vi "Cronometru cu afisaj 7 segmente.vi"() -> ()   [LabVIEW 2011]
panel:
  out "Boolean 46":bool
  out "Boolean 3":bool
  out "Boolean 2":bool
  out "Boolean":bool
  out "Boolean 45":bool
  out "Boolean 44":bool
  out "Boolean 43":bool
  out "Boolean 42":bool
  out "Boolean 41":bool
  out "Boolean 40":bool
  out "Boolean 39":bool
  out "Boolean 38":bool
  out "Boolean 37":bool
  out "Boolean 36":bool
  out "Boolean 35":bool
  out "Boolean 34":bool
  out "Boolean 33":bool
  out "Boolean 32":bool
  out "Boolean 31":bool
  out "Boolean 30":bool
  out "Boolean 29":bool
  out "Boolean 28":bool
  out "Boolean 27":bool
  out "Boolean 26":bool
  out "Boolean 25":bool
  out "Boolean 24":bool
  out "Boolean 23":bool
  out "Boolean 22":bool
  out "Boolean 21":bool
  out "Boolean 20":bool
  out "Boolean 19":bool
  out "Boolean 18":bool
  out "Boolean 17":bool
  out "Boolean 16":bool
  out "Boolean 15":bool
  out "Boolean 14":bool
  out "Boolean 13":bool
  out "Boolean 12":bool
  out "Boolean 11":bool
  out "Boolean 10":bool
  out "Boolean 9":bool
  out "Boolean 8":bool
  out "Boolean 6":bool
  out "Boolean 7":bool
  out "Boolean 5":bool
  out "Boolean 4":bool
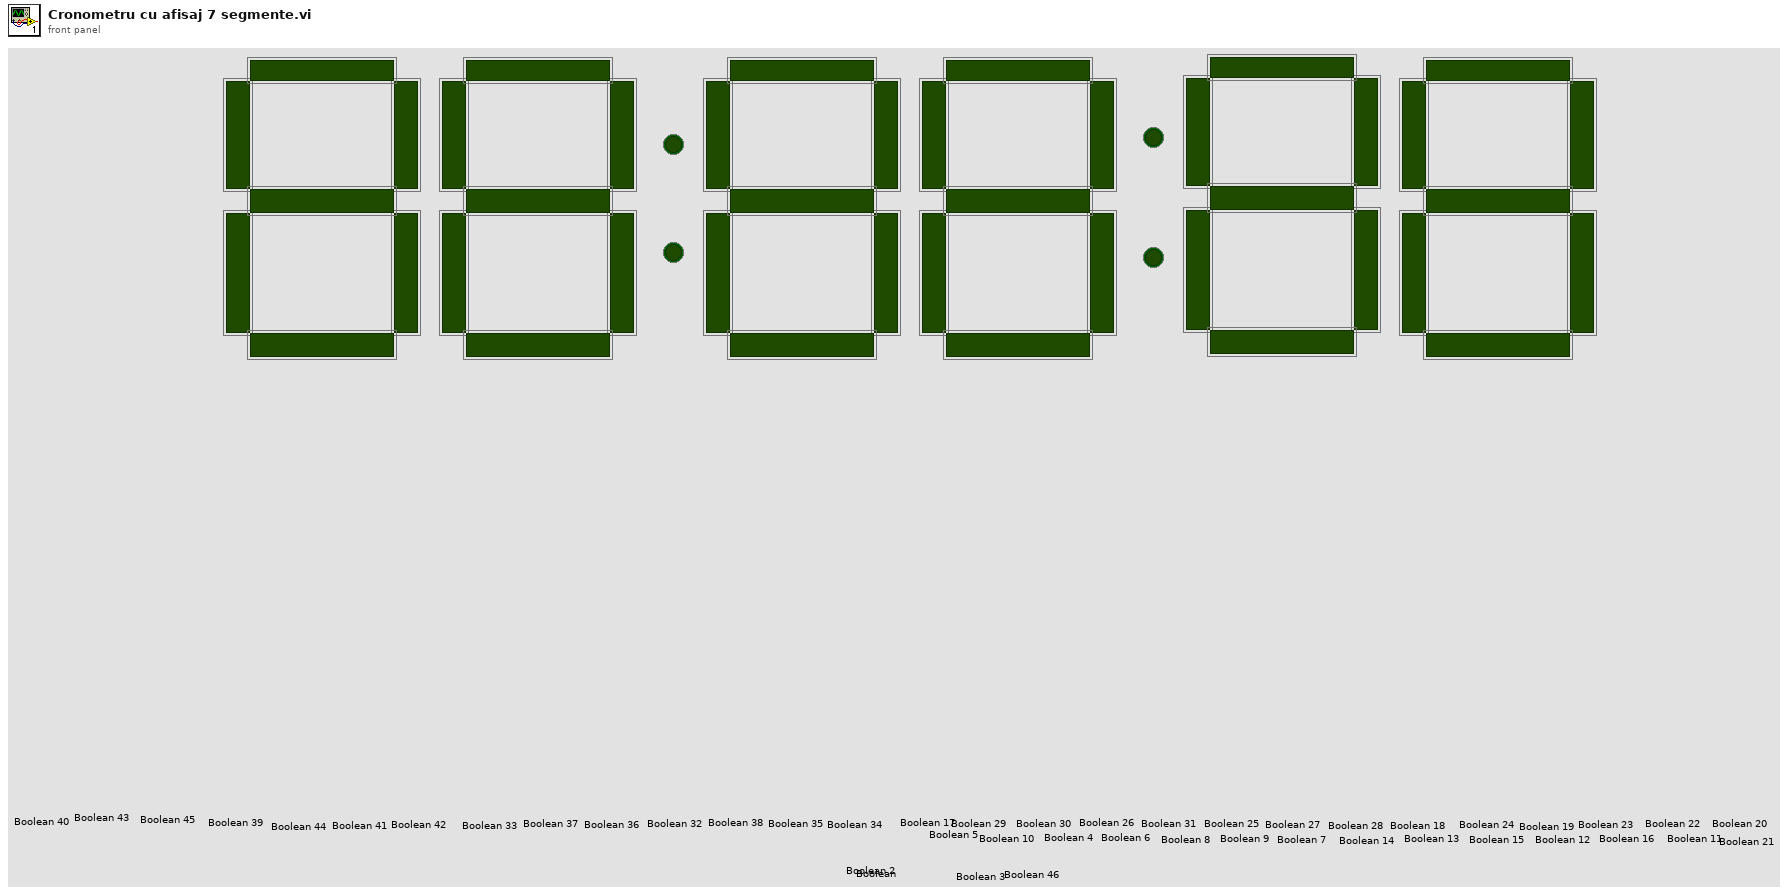
[diagram p1: front panel]
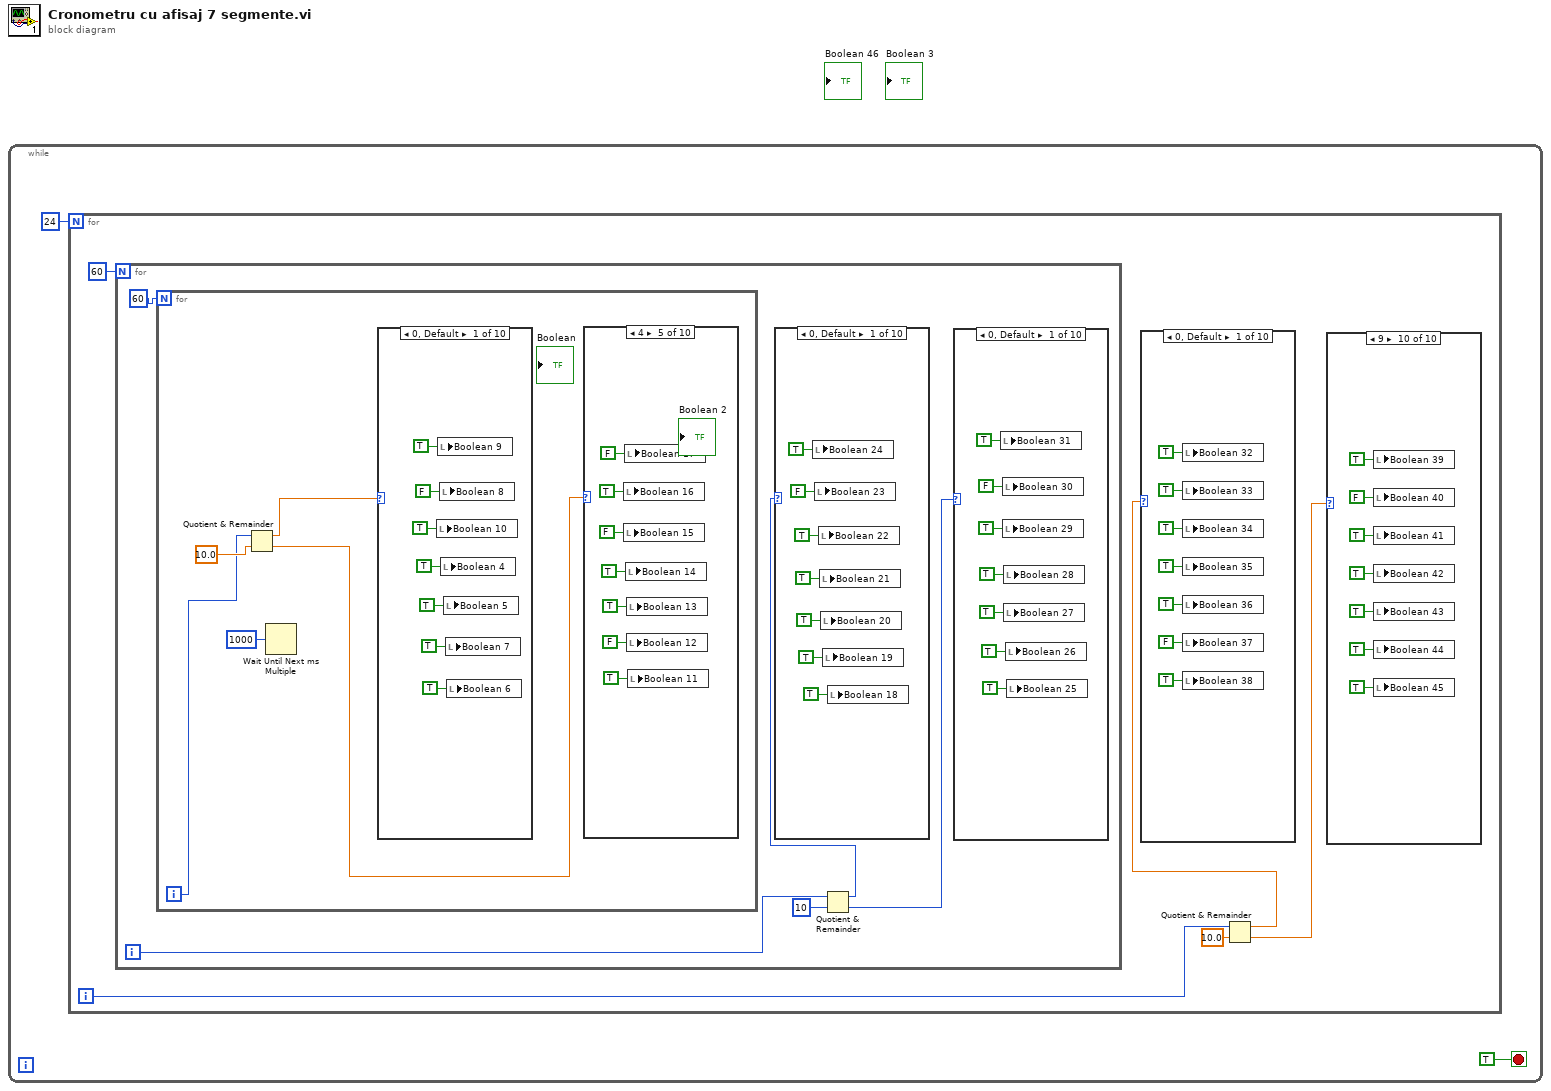
[diagram p0: block diagram]
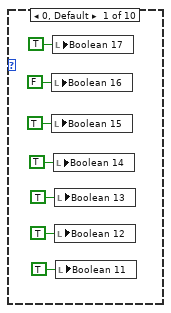
[diagram p2: hidden frame]
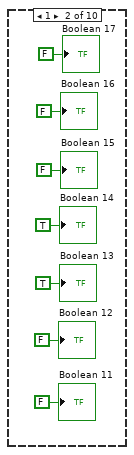
[diagram p3: hidden frame]
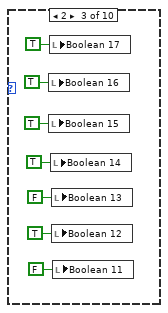
[diagram p4: hidden frame]
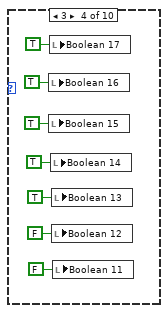
[diagram p5: hidden frame]
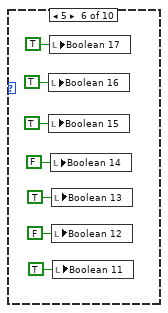
[diagram p6: hidden frame]
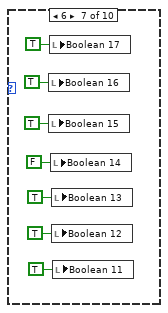
[diagram p7: hidden frame]
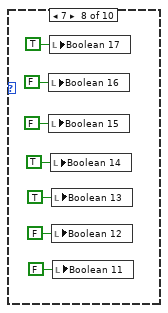
[diagram p8: hidden frame]
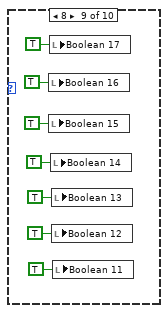
[diagram p9: hidden frame]
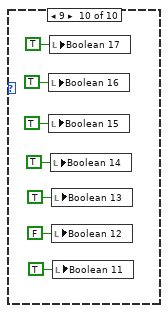
[diagram p10: hidden frame]
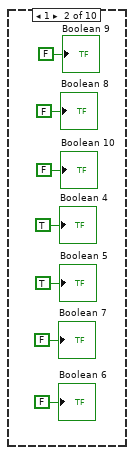
[diagram p11: hidden frame]
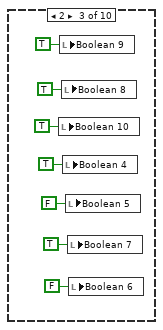
[diagram p12: hidden frame]
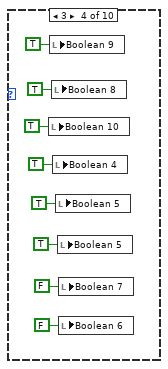
[diagram p13: hidden frame]
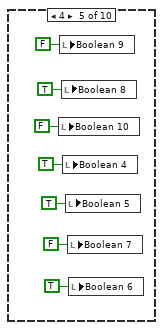
[diagram p14: hidden frame]
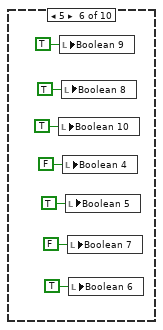
[diagram p15: hidden frame]
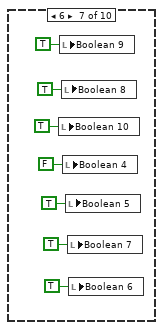
[diagram p16: hidden frame]
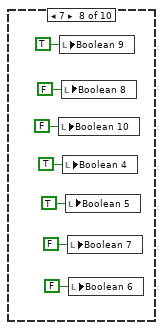
[diagram p17: hidden frame]
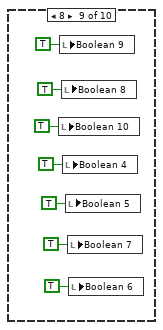
[diagram p18: hidden frame]
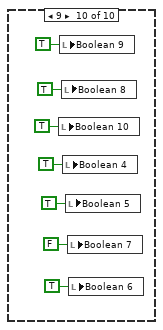
[diagram p19: hidden frame]
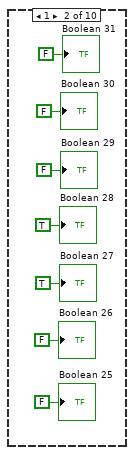
[diagram p20: hidden frame]
diagram:
  n1 = while {
    stop <- TRUE stop-if-true
    n2 = for {
      N: 24 -> [_]
      i -> [w6]
      n3 = for {
        N: 60 -> [_]
        i -> [w11]
        n4 = for {
          N: 60 -> [_]
          i -> [w13]
          n5 = Quotient & Remainder(x=w13, y=10.0 ("x")) -> (x-y*floor(x/y)=w16:dbl, floor(x/y)=w15:dbl)
          n6 = Wait Until Next ms Multiple(millisecond multiple=u32 1000) -> ()  [unwired: 1 out]
          n7 = case shown="0, Default" w16 {
            frame 0, Default {
              n8 = local write "Boolean 10"(TRUE ("Boolean 10")) -> ()
              n9 = local write "Boolean 9"(TRUE ("Boolean 9")) -> ()
              n10 = local write "Boolean 8"(FALSE ("Boolean 8")) -> ()
              n11 = local write "Boolean 4"(TRUE ("Boolean 4")) -> ()
              n12 = local write "Boolean 5"(TRUE ("Boolean 5")) -> ()
              n13 = local write "Boolean 7"(TRUE ("Boolean 5")) -> ()
              n14 = local write "Boolean 6"(TRUE ("Boolean 7")) -> ()
            }
            frame 1 {
              "Boolean 9" <- FALSE ("Boolean 9")
              "Boolean 8" <- FALSE ("Boolean 8")
              "Boolean 10" <- FALSE ("Boolean 10")
              "Boolean 4" <- TRUE ("Boolean 4")
              "Boolean 5" <- TRUE ("Boolean 5")
              "Boolean 7" <- FALSE ("Boolean 7")
              "Boolean 6" <- FALSE ("Boolean 6")
            }
            frame 2 {
              n15 = local write "Boolean 10"(TRUE ("Boolean 10")) -> ()
              n16 = local write "Boolean 9"(TRUE ("Boolean 9")) -> ()
              n17 = local write "Boolean 8"(TRUE ("Boolean 8")) -> ()
              n18 = local write "Boolean 4"(TRUE ("Boolean 4")) -> ()
              n19 = local write "Boolean 5"(FALSE ("Boolean 5")) -> ()
              n20 = local write "Boolean 7"(TRUE ("Boolean 5")) -> ()
              n21 = local write "Boolean 6"(FALSE ("Boolean 7")) -> ()
            }
            frame 3 {
              n22 = local write "Boolean 10"(TRUE ("Boolean 10")) -> ()
              n23 = local write "Boolean 9"(TRUE ("Boolean 9")) -> ()
              n24 = local write "Boolean 8"(TRUE ("Boolean 8")) -> ()
              n25 = local write "Boolean 4"(TRUE ("Boolean 4")) -> ()
              n26 = local write "Boolean 5"(TRUE ("Boolean 5")) -> ()
              n27 = local write "Boolean 5"(TRUE ("Boolean 5")) -> ()
              n28 = local write "Boolean 7"(FALSE ("Boolean 7")) -> ()
              n29 = local write "Boolean 6"(FALSE ("Boolean 6")) -> ()
            }
            frame 4 {
              n30 = local write "Boolean 10"(FALSE ("Boolean 10")) -> ()
              n31 = local write "Boolean 9"(FALSE ("Boolean 9")) -> ()
              n32 = local write "Boolean 8"(TRUE ("Boolean 8")) -> ()
              n33 = local write "Boolean 4"(TRUE ("Boolean 4")) -> ()
              n34 = local write "Boolean 5"(TRUE ("Boolean 5")) -> ()
              n35 = local write "Boolean 7"(FALSE ("Boolean 5")) -> ()
              n36 = local write "Boolean 6"(TRUE ("Boolean 7")) -> ()
            }
            frame 5 {
              n37 = local write "Boolean 10"(TRUE ("Boolean 10")) -> ()
              n38 = local write "Boolean 9"(TRUE ("Boolean 9")) -> ()
              n39 = local write "Boolean 8"(TRUE ("Boolean 8")) -> ()
              n40 = local write "Boolean 4"(FALSE ("Boolean 4")) -> ()
              n41 = local write "Boolean 5"(TRUE ("Boolean 5")) -> ()
              n42 = local write "Boolean 7"(FALSE ("Boolean 5")) -> ()
              n43 = local write "Boolean 6"(TRUE ("Boolean 7")) -> ()
            }
            frame 6 {
              n44 = local write "Boolean 10"(TRUE ("Boolean 10")) -> ()
              n45 = local write "Boolean 9"(TRUE ("Boolean 9")) -> ()
              n46 = local write "Boolean 8"(TRUE ("Boolean 8")) -> ()
              n47 = local write "Boolean 4"(FALSE ("Boolean 4")) -> ()
              n48 = local write "Boolean 5"(TRUE ("Boolean 5")) -> ()
              n49 = local write "Boolean 7"(TRUE ("Boolean 5")) -> ()
              n50 = local write "Boolean 6"(TRUE ("Boolean 7")) -> ()
            }
            frame 7 {
              n51 = local write "Boolean 10"(FALSE ("Boolean 10")) -> ()
              n52 = local write "Boolean 9"(TRUE ("Boolean 9")) -> ()
              n53 = local write "Boolean 8"(FALSE ("Boolean 8")) -> ()
              n54 = local write "Boolean 4"(TRUE ("Boolean 4")) -> ()
              n55 = local write "Boolean 5"(TRUE ("Boolean 5")) -> ()
              n56 = local write "Boolean 7"(FALSE ("Boolean 5")) -> ()
              n57 = local write "Boolean 6"(FALSE ("Boolean 7")) -> ()
            }
            frame 8 {
              n58 = local write "Boolean 10"(TRUE ("Boolean 10")) -> ()
              n59 = local write "Boolean 9"(TRUE ("Boolean 9")) -> ()
              n60 = local write "Boolean 8"(TRUE ("Boolean 8")) -> ()
              n61 = local write "Boolean 4"(TRUE ("Boolean 4")) -> ()
              n62 = local write "Boolean 5"(TRUE ("Boolean 5")) -> ()
              n63 = local write "Boolean 7"(TRUE ("Boolean 5")) -> ()
              n64 = local write "Boolean 6"(TRUE ("Boolean 7")) -> ()
            }
            frame 9 {
              n65 = local write "Boolean 10"(TRUE ("Boolean 10")) -> ()
              n66 = local write "Boolean 9"(TRUE ("Boolean 9")) -> ()
              n67 = local write "Boolean 8"(TRUE ("Boolean 8")) -> ()
              n68 = local write "Boolean 4"(TRUE ("Boolean 4")) -> ()
              n69 = local write "Boolean 5"(TRUE ("Boolean 5")) -> ()
              n70 = local write "Boolean 7"(FALSE ("Boolean 5")) -> ()
              n71 = local write "Boolean 6"(TRUE ("Boolean 7")) -> ()
            }
          }
          n72 = case shown="4" w15 {
            frame 0, Default {
              n73 = local write "Boolean 16"(FALSE ("Boolean 16")) -> ()
              n74 = local write "Boolean 15"(TRUE ("Boolean 15")) -> ()
              n75 = local write "Boolean 17"(TRUE ("Boolean 17")) -> ()
              n76 = local write "Boolean 14"(TRUE ("Boolean 14")) -> ()
              n77 = local write "Boolean 13"(TRUE ("Boolean 13")) -> ()
              n78 = local write "Boolean 12"(TRUE ("Boolean 12")) -> ()
              n79 = local write "Boolean 11"(TRUE ("Boolean 11")) -> ()
            }
            frame 1 {
              "Boolean 17" <- FALSE ("Boolean 9")
              "Boolean 16" <- FALSE ("Boolean 8")
              "Boolean 15" <- FALSE ("Boolean 10")
              "Boolean 14" <- TRUE ("Boolean 4")
              "Boolean 13" <- TRUE ("Boolean 5")
              "Boolean 12" <- FALSE ("Boolean 7")
              "Boolean 11" <- FALSE ("Boolean 6")
            }
            frame 2 {
              n80 = local write "Boolean 16"(TRUE ("Boolean 16")) -> ()
              n81 = local write "Boolean 15"(TRUE ("Boolean 15")) -> ()
              n82 = local write "Boolean 17"(TRUE ("Boolean 17")) -> ()
              n83 = local write "Boolean 14"(TRUE ("Boolean 14")) -> ()
              n84 = local write "Boolean 13"(FALSE ("Boolean 13")) -> ()
              n85 = local write "Boolean 12"(TRUE ("Boolean 12")) -> ()
              n86 = local write "Boolean 11"(FALSE ("Boolean 11")) -> ()
            }
            frame 3 {
              n87 = local write "Boolean 16"(TRUE ("Boolean 16")) -> ()
              n88 = local write "Boolean 15"(TRUE ("Boolean 15")) -> ()
              n89 = local write "Boolean 17"(TRUE ("Boolean 17")) -> ()
              n90 = local write "Boolean 14"(TRUE ("Boolean 14")) -> ()
              n91 = local write "Boolean 13"(TRUE ("Boolean 13")) -> ()
              n92 = local write "Boolean 12"(FALSE ("Boolean 12")) -> ()
              n93 = local write "Boolean 11"(FALSE ("Boolean 11")) -> ()
            }
            frame 4 {
              n94 = local write "Boolean 16"(TRUE ("Boolean 16")) -> ()
              n95 = local write "Boolean 15"(FALSE ("Boolean 15")) -> ()
              n96 = local write "Boolean 17"(FALSE ("Boolean 17")) -> ()
              n97 = local write "Boolean 14"(TRUE ("Boolean 14")) -> ()
              n98 = local write "Boolean 13"(TRUE ("Boolean 13")) -> ()
              n99 = local write "Boolean 12"(FALSE ("Boolean 12")) -> ()
              n100 = local write "Boolean 11"(TRUE ("Boolean 11")) -> ()
            }
            frame 5 {
              n101 = local write "Boolean 16"(TRUE ("Boolean 16")) -> ()
              n102 = local write "Boolean 15"(TRUE ("Boolean 15")) -> ()
              n103 = local write "Boolean 17"(TRUE ("Boolean 17")) -> ()
              n104 = local write "Boolean 14"(FALSE ("Boolean 14")) -> ()
              n105 = local write "Boolean 13"(TRUE ("Boolean 13")) -> ()
              n106 = local write "Boolean 12"(FALSE ("Boolean 12")) -> ()
              n107 = local write "Boolean 11"(TRUE ("Boolean 11")) -> ()
            }
            frame 6 {
              n108 = local write "Boolean 16"(TRUE ("Boolean 16")) -> ()
              n109 = local write "Boolean 15"(TRUE ("Boolean 15")) -> ()
              n110 = local write "Boolean 17"(TRUE ("Boolean 17")) -> ()
              n111 = local write "Boolean 14"(FALSE ("Boolean 14")) -> ()
              n112 = local write "Boolean 13"(TRUE ("Boolean 13")) -> ()
              n113 = local write "Boolean 12"(TRUE ("Boolean 12")) -> ()
              n114 = local write "Boolean 11"(TRUE ("Boolean 11")) -> ()
            }
            frame 7 {
              n115 = local write "Boolean 16"(FALSE ("Boolean 16")) -> ()
              n116 = local write "Boolean 15"(FALSE ("Boolean 15")) -> ()
              n117 = local write "Boolean 17"(TRUE ("Boolean 17")) -> ()
              n118 = local write "Boolean 14"(TRUE ("Boolean 14")) -> ()
              n119 = local write "Boolean 13"(TRUE ("Boolean 13")) -> ()
              n120 = local write "Boolean 12"(FALSE ("Boolean 12")) -> ()
              n121 = local write "Boolean 11"(FALSE ("Boolean 11")) -> ()
            }
            frame 8 {
              n122 = local write "Boolean 16"(TRUE ("Boolean 16")) -> ()
              n123 = local write "Boolean 15"(TRUE ("Boolean 15")) -> ()
              n124 = local write "Boolean 17"(TRUE ("Boolean 17")) -> ()
              n125 = local write "Boolean 14"(TRUE ("Boolean 14")) -> ()
              n126 = local write "Boolean 13"(TRUE ("Boolean 13")) -> ()
              n127 = local write "Boolean 12"(TRUE ("Boolean 12")) -> ()
              n128 = local write "Boolean 11"(TRUE ("Boolean 11")) -> ()
            }
            frame 9 {
              n129 = local write "Boolean 16"(TRUE ("Boolean 16")) -> ()
              n130 = local write "Boolean 15"(TRUE ("Boolean 15")) -> ()
              n131 = local write "Boolean 17"(TRUE ("Boolean 17")) -> ()
              n132 = local write "Boolean 14"(TRUE ("Boolean 14")) -> ()
              n133 = local write "Boolean 13"(TRUE ("Boolean 13")) -> ()
              n134 = local write "Boolean 12"(FALSE ("Boolean 12")) -> ()
              n135 = local write "Boolean 11"(TRUE ("Boolean 11")) -> ()
            }
          }
        }
        n136 = Quotient & Remainder(x=w11, y=10) -> (x-y*floor(x/y)=w9:i32, floor(x/y)=w8:i32)
        n137 = case shown="0, Default" w9 {
          frame 0, Default {
            n138 = local write "Boolean 24"(TRUE ("Boolean 24")) -> ()
            n139 = local write "Boolean 23"(FALSE ("Boolean 23")) -> ()
            n140 = local write "Boolean 22"(TRUE ("Boolean 22")) -> ()
            n141 = local write "Boolean 21"(TRUE ("Boolean 21")) -> ()
            n142 = local write "Boolean 20"(TRUE ("Boolean 20")) -> ()
            n143 = local write "Boolean 19"(TRUE ("Boolean 19")) -> ()
            n144 = local write "Boolean 18"(TRUE ("Boolean 18")) -> ()
          }
          frame 1 {
            "Boolean 24" <- FALSE ("Boolean 9")
            "Boolean 23" <- FALSE ("Boolean 8")
            "Boolean 22" <- FALSE ("Boolean 10")
            "Boolean 21" <- TRUE ("Boolean 4")
            "Boolean 20" <- TRUE ("Boolean 5")
            "Boolean 19" <- FALSE ("Boolean 7")
            "Boolean 18" <- FALSE ("Boolean 6")
          }
          frame 2 {
            n145 = local write "Boolean 24"(TRUE ("Boolean 24")) -> ()
            n146 = local write "Boolean 23"(TRUE ("Boolean 23")) -> ()
            n147 = local write "Boolean 22"(TRUE ("Boolean 22")) -> ()
            n148 = local write "Boolean 21"(TRUE ("Boolean 21")) -> ()
            n149 = local write "Boolean 20"(FALSE ("Boolean 20")) -> ()
            n150 = local write "Boolean 19"(TRUE ("Boolean 19")) -> ()
            n151 = local write "Boolean 18"(FALSE ("Boolean 18")) -> ()
          }
          frame 3 {
            n152 = local write "Boolean 24"(TRUE ("Boolean 24")) -> ()
            n153 = local write "Boolean 23"(TRUE ("Boolean 23")) -> ()
            n154 = local write "Boolean 22"(TRUE ("Boolean 22")) -> ()
            n155 = local write "Boolean 21"(TRUE ("Boolean 21")) -> ()
            n156 = local write "Boolean 20"(TRUE ("Boolean 20")) -> ()
            n157 = local write "Boolean 19"(FALSE ("Boolean 19")) -> ()
            n158 = local write "Boolean 18"(FALSE ("Boolean 18")) -> ()
          }
          frame 4 {
            n159 = local write "Boolean 24"(FALSE ("Boolean 24")) -> ()
            n160 = local write "Boolean 23"(TRUE ("Boolean 23")) -> ()
            n161 = local write "Boolean 22"(FALSE ("Boolean 22")) -> ()
            n162 = local write "Boolean 21"(TRUE ("Boolean 21")) -> ()
            n163 = local write "Boolean 20"(TRUE ("Boolean 20")) -> ()
            n164 = local write "Boolean 19"(FALSE ("Boolean 19")) -> ()
            n165 = local write "Boolean 18"(TRUE ("Boolean 18")) -> ()
          }
          frame 5 {
            n166 = local write "Boolean 24"(TRUE ("Boolean 24")) -> ()
            n167 = local write "Boolean 23"(TRUE ("Boolean 23")) -> ()
            n168 = local write "Boolean 22"(TRUE ("Boolean 22")) -> ()
            n169 = local write "Boolean 21"(FALSE ("Boolean 21")) -> ()
            n170 = local write "Boolean 20"(TRUE ("Boolean 20")) -> ()
            n171 = local write "Boolean 19"(FALSE ("Boolean 19")) -> ()
            n172 = local write "Boolean 18"(TRUE ("Boolean 18")) -> ()
          }
          frame 6 {
            n173 = local write "Boolean 24"(TRUE ("Boolean 24")) -> ()
            n174 = local write "Boolean 23"(TRUE ("Boolean 23")) -> ()
            n175 = local write "Boolean 22"(TRUE ("Boolean 22")) -> ()
            n176 = local write "Boolean 21"(FALSE ("Boolean 21")) -> ()
            n177 = local write "Boolean 20"(TRUE ("Boolean 20")) -> ()
            n178 = local write "Boolean 19"(TRUE ("Boolean 19")) -> ()
            n179 = local write "Boolean 18"(TRUE ("Boolean 18")) -> ()
          }
          frame 7 {
            n180 = local write "Boolean 24"(TRUE ("Boolean 24")) -> ()
            n181 = local write "Boolean 23"(FALSE ("Boolean 23")) -> ()
            n182 = local write "Boolean 22"(FALSE ("Boolean 22")) -> ()
            n183 = local write "Boolean 21"(TRUE ("Boolean 21")) -> ()
            n184 = local write "Boolean 20"(TRUE ("Boolean 20")) -> ()
            n185 = local write "Boolean 19"(FALSE ("Boolean 19")) -> ()
            n186 = local write "Boolean 18"(FALSE ("Boolean 18")) -> ()
          }
          frame 8 {
            n187 = local write "Boolean 24"(TRUE ("Boolean 24")) -> ()
            n188 = local write "Boolean 23"(TRUE ("Boolean 23")) -> ()
            n189 = local write "Boolean 22"(TRUE ("Boolean 22")) -> ()
            n190 = local write "Boolean 21"(TRUE ("Boolean 21")) -> ()
            n191 = local write "Boolean 20"(TRUE ("Boolean 20")) -> ()
            n192 = local write "Boolean 19"(TRUE ("Boolean 19")) -> ()
            n193 = local write "Boolean 18"(TRUE ("Boolean 18")) -> ()
          }
          frame 9 {
            n194 = local write "Boolean 24"(TRUE ("Boolean 24")) -> ()
            n195 = local write "Boolean 23"(TRUE ("Boolean 23")) -> ()
            n196 = local write "Boolean 22"(TRUE ("Boolean 22")) -> ()
            n197 = local write "Boolean 21"(TRUE ("Boolean 21")) -> ()
            n198 = local write "Boolean 20"(TRUE ("Boolean 20")) -> ()
            n199 = local write "Boolean 19"(FALSE ("Boolean 19")) -> ()
            n200 = local write "Boolean 18"(TRUE ("Boolean 18")) -> ()
          }
        }
        n201 = case shown="0, Default" w8 {
          frame 0, Default {
            n202 = local write "Boolean 31"(TRUE ("Boolean 31")) -> ()
            n203 = local write "Boolean 30"(FALSE ("Boolean 30")) -> ()
            n204 = local write "Boolean 29"(TRUE ("Boolean 29")) -> ()
            n205 = local write "Boolean 28"(TRUE ("Boolean 28")) -> ()
            n206 = local write "Boolean 27"(TRUE ("Boolean 27")) -> ()
            n207 = local write "Boolean 26"(TRUE ("Boolean 26")) -> ()
            n208 = local write "Boolean 25"(TRUE ("Boolean 25")) -> ()
          }
          frame 1 {
            "Boolean 31" <- FALSE ("Boolean 9")
            "Boolean 30" <- FALSE ("Boolean 8")
            "Boolean 29" <- FALSE ("Boolean 10")
            "Boolean 28" <- TRUE ("Boolean 4")
            "Boolean 27" <- TRUE ("Boolean 5")
            "Boolean 26" <- FALSE ("Boolean 7")
            "Boolean 25" <- FALSE ("Boolean 6")
          }
          frame 2 {
            n209 = local write "Boolean 31"(TRUE ("Boolean 31")) -> ()
            n210 = local write "Boolean 30"(TRUE ("Boolean 30")) -> ()
            n211 = local write "Boolean 29"(TRUE ("Boolean 29")) -> ()
            n212 = local write "Boolean 28"(TRUE ("Boolean 28")) -> ()
            n213 = local write "Boolean 27"(FALSE ("Boolean 27")) -> ()
            n214 = local write "Boolean 26"(TRUE ("Boolean 26")) -> ()
            n215 = local write "Boolean 25"(FALSE ("Boolean 25")) -> ()
          }
          frame 3 {
            n216 = local write "Boolean 31"(TRUE ("Boolean 31")) -> ()
            n217 = local write "Boolean 30"(TRUE ("Boolean 30")) -> ()
            n218 = local write "Boolean 29"(TRUE ("Boolean 29")) -> ()
            n219 = local write "Boolean 28"(TRUE ("Boolean 28")) -> ()
            n220 = local write "Boolean 27"(TRUE ("Boolean 27")) -> ()
            n221 = local write "Boolean 26"(FALSE ("Boolean 26")) -> ()
            n222 = local write "Boolean 25"(FALSE ("Boolean 25")) -> ()
          }
          frame 4 {
            n223 = local write "Boolean 31"(FALSE ("Boolean 31")) -> ()
            n224 = local write "Boolean 30"(TRUE ("Boolean 30")) -> ()
            n225 = local write "Boolean 29"(FALSE ("Boolean 29")) -> ()
            n226 = local write "Boolean 28"(TRUE ("Boolean 28")) -> ()
            n227 = local write "Boolean 27"(TRUE ("Boolean 27")) -> ()
            n228 = local write "Boolean 26"(FALSE ("Boolean 26")) -> ()
            n229 = local write "Boolean 25"(TRUE ("Boolean 25")) -> ()
          }
          frame 5 {
            n230 = local write "Boolean 31"(TRUE ("Boolean 31")) -> ()
            n231 = local write "Boolean 30"(TRUE ("Boolean 30")) -> ()
            n232 = local write "Boolean 29"(TRUE ("Boolean 29")) -> ()
            n233 = local write "Boolean 28"(FALSE ("Boolean 28")) -> ()
            n234 = local write "Boolean 27"(TRUE ("Boolean 27")) -> ()
            n235 = local write "Boolean 26"(FALSE ("Boolean 26")) -> ()
            n236 = local write "Boolean 25"(TRUE ("Boolean 25")) -> ()
          }
          frame 6 {
            n237 = local write "Boolean 31"(TRUE ("Boolean 31")) -> ()
            n238 = local write "Boolean 30"(TRUE ("Boolean 30")) -> ()
            n239 = local write "Boolean 29"(TRUE ("Boolean 29")) -> ()
            n240 = local write "Boolean 28"(FALSE ("Boolean 28")) -> ()
            n241 = local write "Boolean 27"(TRUE ("Boolean 27")) -> ()
            n242 = local write "Boolean 26"(TRUE ("Boolean 26")) -> ()
            n243 = local write "Boolean 25"(TRUE ("Boolean 25")) -> ()
          }
          frame 7 {
            n244 = local write "Boolean 31"(TRUE ("Boolean 31")) -> ()
            n245 = local write "Boolean 30"(FALSE ("Boolean 30")) -> ()
            n246 = local write "Boolean 29"(FALSE ("Boolean 29")) -> ()
            n247 = local write "Boolean 28"(TRUE ("Boolean 28")) -> ()
            n248 = local write "Boolean 27"(TRUE ("Boolean 27")) -> ()
            n249 = local write "Boolean 26"(FALSE ("Boolean 26")) -> ()
            n250 = local write "Boolean 25"(FALSE ("Boolean 25")) -> ()
          }
          frame 8 {
            n251 = local write "Boolean 31"(TRUE ("Boolean 31")) -> ()
            n252 = local write "Boolean 30"(TRUE ("Boolean 30")) -> ()
            n253 = local write "Boolean 29"(TRUE ("Boolean 29")) -> ()
            n254 = local write "Boolean 28"(TRUE ("Boolean 28")) -> ()
            n255 = local write "Boolean 27"(TRUE ("Boolean 27")) -> ()
            n256 = local write "Boolean 26"(TRUE ("Boolean 26")) -> ()
            n257 = local write "Boolean 25"(TRUE ("Boolean 25")) -> ()
          }
          frame 9 {
            n258 = local write "Boolean 31"(TRUE ("Boolean 31")) -> ()
            n259 = local write "Boolean 30"(TRUE ("Boolean 30")) -> ()
            n260 = local write "Boolean 29"(TRUE ("Boolean 29")) -> ()
            n261 = local write "Boolean 28"(TRUE ("Boolean 28")) -> ()
            n262 = local write "Boolean 27"(TRUE ("Boolean 27")) -> ()
            n263 = local write "Boolean 26"(FALSE ("Boolean 26")) -> ()
            n264 = local write "Boolean 25"(TRUE ("Boolean 25")) -> ()
          }
        }
      }
      n265 = Quotient & Remainder(x=w6, y=10.0 ("floor(x/y)")) -> (x-y*floor(x/y)=w5:dbl, floor(x/y)=w4:dbl)
      n266 = case shown="0, Default" w5 {
        frame 0, Default {
          n267 = local write "Boolean 32"(TRUE ("Boolean 32")) -> ()
          n268 = local write "Boolean 33"(TRUE ("Boolean 33")) -> ()
          n269 = local write "Boolean 34"(TRUE ("Boolean 34")) -> ()
          n270 = local write "Boolean 35"(TRUE ("Boolean 35")) -> ()
          n271 = local write "Boolean 36"(TRUE ("Boolean 36")) -> ()
          n272 = local write "Boolean 37"(FALSE ("Boolean 37")) -> ()
          n273 = local write "Boolean 38"(TRUE ("Boolean 38")) -> ()
        }
        frame 1 {
          "Boolean 38" <- FALSE ("Boolean 9")
          "Boolean 37" <- FALSE ("Boolean 8")
          "Boolean 36" <- FALSE ("Boolean 10")
          "Boolean 35" <- TRUE ("Boolean 4")
          "Boolean 34" <- TRUE ("Boolean 5")
          "Boolean 33" <- FALSE ("Boolean 7")
          "Boolean 32" <- FALSE ("Boolean 6")
        }
        frame 2 {
          n274 = local write "Boolean 32"(FALSE ("Boolean 32")) -> ()
          n275 = local write "Boolean 33"(TRUE ("Boolean 33")) -> ()
          n276 = local write "Boolean 34"(FALSE ("Boolean 34")) -> ()
          n277 = local write "Boolean 35"(TRUE ("Boolean 35")) -> ()
          n278 = local write "Boolean 36"(TRUE ("Boolean 36")) -> ()
          n279 = local write "Boolean 37"(TRUE ("Boolean 37")) -> ()
          n280 = local write "Boolean 38"(TRUE ("Boolean 38")) -> ()
        }
        frame 3 {
          n281 = local write "Boolean 32"(FALSE ("Boolean 32")) -> ()
          n282 = local write "Boolean 33"(FALSE ("Boolean 33")) -> ()
          n283 = local write "Boolean 34"(TRUE ("Boolean 34")) -> ()
          n284 = local write "Boolean 35"(TRUE ("Boolean 35")) -> ()
          n285 = local write "Boolean 36"(TRUE ("Boolean 36")) -> ()
          n286 = local write "Boolean 37"(TRUE ("Boolean 37")) -> ()
          n287 = local write "Boolean 38"(TRUE ("Boolean 38")) -> ()
        }
        frame 4 {
          n288 = local write "Boolean 32"(TRUE ("Boolean 32")) -> ()
          n289 = local write "Boolean 33"(FALSE ("Boolean 33")) -> ()
          n290 = local write "Boolean 34"(TRUE ("Boolean 34")) -> ()
          n291 = local write "Boolean 35"(TRUE ("Boolean 35")) -> ()
          n292 = local write "Boolean 36"(FALSE ("Boolean 36")) -> ()
          n293 = local write "Boolean 37"(TRUE ("Boolean 37")) -> ()
          n294 = local write "Boolean 38"(FALSE ("Boolean 38")) -> ()
        }
        frame 5 {
          n295 = local write "Boolean 32"(TRUE ("Boolean 32")) -> ()
          n296 = local write "Boolean 33"(FALSE ("Boolean 33")) -> ()
          n297 = local write "Boolean 34"(TRUE ("Boolean 34")) -> ()
          n298 = local write "Boolean 35"(FALSE ("Boolean 35")) -> ()
          n299 = local write "Boolean 36"(TRUE ("Boolean 36")) -> ()
          n300 = local write "Boolean 37"(TRUE ("Boolean 37")) -> ()
          n301 = local write "Boolean 38"(TRUE ("Boolean 38")) -> ()
        }
        frame 6 {
          n302 = local write "Boolean 32"(TRUE ("Boolean 32")) -> ()
          n303 = local write "Boolean 33"(TRUE ("Boolean 33")) -> ()
          n304 = local write "Boolean 34"(TRUE ("Boolean 34")) -> ()
          n305 = local write "Boolean 35"(FALSE ("Boolean 35")) -> ()
          n306 = local write "Boolean 36"(TRUE ("Boolean 36")) -> ()
          n307 = local write "Boolean 37"(TRUE ("Boolean 37")) -> ()
          n308 = local write "Boolean 38"(TRUE ("Boolean 38")) -> ()
        }
        frame 7 {
          n309 = local write "Boolean 32"(FALSE ("Boolean 32")) -> ()
          n310 = local write "Boolean 33"(FALSE ("Boolean 33")) -> ()
          n311 = local write "Boolean 34"(TRUE ("Boolean 34")) -> ()
          n312 = local write "Boolean 35"(TRUE ("Boolean 35")) -> ()
          n313 = local write "Boolean 36"(FALSE ("Boolean 36")) -> ()
          n314 = local write "Boolean 37"(FALSE ("Boolean 37")) -> ()
          n315 = local write "Boolean 38"(TRUE ("Boolean 38")) -> ()
        }
        frame 8 {
          n316 = local write "Boolean 32"(TRUE ("Boolean 32")) -> ()
          n317 = local write "Boolean 33"(TRUE ("Boolean 33")) -> ()
          n318 = local write "Boolean 34"(TRUE ("Boolean 34")) -> ()
          n319 = local write "Boolean 35"(TRUE ("Boolean 35")) -> ()
          n320 = local write "Boolean 36"(TRUE ("Boolean 36")) -> ()
          n321 = local write "Boolean 37"(TRUE ("Boolean 37")) -> ()
          n322 = local write "Boolean 38"(TRUE ("Boolean 38")) -> ()
        }
        frame 9 {
          n323 = local write "Boolean 32"(TRUE ("Boolean 32")) -> ()
          n324 = local write "Boolean 33"(FALSE ("Boolean 33")) -> ()
          n325 = local write "Boolean 34"(TRUE ("Boolean 34")) -> ()
          n326 = local write "Boolean 35"(TRUE ("Boolean 35")) -> ()
          n327 = local write "Boolean 36"(TRUE ("Boolean 36")) -> ()
          n328 = local write "Boolean 37"(TRUE ("Boolean 37")) -> ()
          n329 = local write "Boolean 38"(TRUE ("Boolean 38")) -> ()
        }
      }
      n330 = case shown="9" w4 {
        frame 0, Default {
          n331 = local write "Boolean 39"(TRUE ("Boolean 39")) -> ()
          n332 = local write "Boolean 40"(TRUE ("Boolean 40")) -> ()
          n333 = local write "Boolean 41"(TRUE ("Boolean 41")) -> ()
          n334 = local write "Boolean 42"(TRUE ("Boolean 42")) -> ()
          n335 = local write "Boolean 43"(TRUE ("Boolean 43")) -> ()
          n336 = local write "Boolean 44"(FALSE ("Boolean 44")) -> ()
          n337 = local write "Boolean 45"(TRUE ("Boolean 45")) -> ()
        }
        frame 1 {
          "Boolean 45" <- FALSE ("Boolean 9")
          "Boolean 44" <- FALSE ("Boolean 8")
          "Boolean 43" <- FALSE ("Boolean 10")
          "Boolean 42" <- TRUE ("Boolean 4")
          "Boolean 41" <- TRUE ("Boolean 5")
          "Boolean 40" <- FALSE ("Boolean 7")
          "Boolean 39" <- FALSE ("Boolean 6")
        }
        frame 2 {
          n338 = local write "Boolean 39"(FALSE ("Boolean 39")) -> ()
          n339 = local write "Boolean 40"(TRUE ("Boolean 40")) -> ()
          n340 = local write "Boolean 41"(FALSE ("Boolean 41")) -> ()
          n341 = local write "Boolean 42"(TRUE ("Boolean 42")) -> ()
          n342 = local write "Boolean 43"(TRUE ("Boolean 43")) -> ()
          n343 = local write "Boolean 44"(TRUE ("Boolean 44")) -> ()
          n344 = local write "Boolean 45"(TRUE ("Boolean 45")) -> ()
        }
        frame 3 {
          n345 = local write "Boolean 39"(FALSE ("Boolean 39")) -> ()
          n346 = local write "Boolean 40"(FALSE ("Boolean 40")) -> ()
          n347 = local write "Boolean 41"(TRUE ("Boolean 41")) -> ()
          n348 = local write "Boolean 42"(TRUE ("Boolean 42")) -> ()
          n349 = local write "Boolean 43"(TRUE ("Boolean 43")) -> ()
          n350 = local write "Boolean 44"(TRUE ("Boolean 44")) -> ()
          n351 = local write "Boolean 45"(TRUE ("Boolean 45")) -> ()
        }
        frame 4 {
          n352 = local write "Boolean 39"(TRUE ("Boolean 39")) -> ()
          n353 = local write "Boolean 40"(FALSE ("Boolean 40")) -> ()
          n354 = local write "Boolean 41"(TRUE ("Boolean 41")) -> ()
          n355 = local write "Boolean 42"(TRUE ("Boolean 42")) -> ()
          n356 = local write "Boolean 43"(FALSE ("Boolean 43")) -> ()
          n357 = local write "Boolean 44"(TRUE ("Boolean 44")) -> ()
          n358 = local write "Boolean 45"(FALSE ("Boolean 45")) -> ()
        }
        frame 5 {
          n359 = local write "Boolean 39"(TRUE ("Boolean 39")) -> ()
          n360 = local write "Boolean 40"(FALSE ("Boolean 40")) -> ()
          n361 = local write "Boolean 41"(TRUE ("Boolean 41")) -> ()
          n362 = local write "Boolean 42"(FALSE ("Boolean 42")) -> ()
          n363 = local write "Boolean 43"(TRUE ("Boolean 43")) -> ()
          n364 = local write "Boolean 44"(TRUE ("Boolean 44")) -> ()
          n365 = local write "Boolean 45"(TRUE ("Boolean 45")) -> ()
        }
        frame 6 {
          n366 = local write "Boolean 39"(TRUE ("Boolean 39")) -> ()
          n367 = local write "Boolean 40"(TRUE ("Boolean 40")) -> ()
          n368 = local write "Boolean 41"(TRUE ("Boolean 41")) -> ()
          n369 = local write "Boolean 42"(FALSE ("Boolean 42")) -> ()
          n370 = local write "Boolean 43"(TRUE ("Boolean 43")) -> ()
          n371 = local write "Boolean 44"(TRUE ("Boolean 44")) -> ()
          n372 = local write "Boolean 45"(TRUE ("Boolean 45")) -> ()
        }
        frame 7 {
          n373 = local write "Boolean 39"(FALSE ("Boolean 39")) -> ()
          n374 = local write "Boolean 40"(FALSE ("Boolean 40")) -> ()
          n375 = local write "Boolean 41"(TRUE ("Boolean 41")) -> ()
          n376 = local write "Boolean 42"(TRUE ("Boolean 42")) -> ()
          n377 = local write "Boolean 43"(FALSE ("Boolean 43")) -> ()
          n378 = local write "Boolean 44"(FALSE ("Boolean 44")) -> ()
          n379 = local write "Boolean 45"(TRUE ("Boolean 45")) -> ()
        }
        frame 8 {
          n380 = local write "Boolean 39"(TRUE ("Boolean 39")) -> ()
          n381 = local write "Boolean 40"(TRUE ("Boolean 40")) -> ()
          n382 = local write "Boolean 41"(TRUE ("Boolean 41")) -> ()
          n383 = local write "Boolean 42"(TRUE ("Boolean 42")) -> ()
          n384 = local write "Boolean 43"(TRUE ("Boolean 43")) -> ()
          n385 = local write "Boolean 44"(TRUE ("Boolean 44")) -> ()
          n386 = local write "Boolean 45"(TRUE ("Boolean 45")) -> ()
        }
        frame 9 {
          n387 = local write "Boolean 39"(TRUE ("Boolean 39")) -> ()
          n388 = local write "Boolean 40"(FALSE ("Boolean 40")) -> ()
          n389 = local write "Boolean 41"(TRUE ("Boolean 41")) -> ()
          n390 = local write "Boolean 42"(TRUE ("Boolean 42")) -> ()
          n391 = local write "Boolean 43"(TRUE ("Boolean 43")) -> ()
          n392 = local write "Boolean 44"(TRUE ("Boolean 44")) -> ()
          n393 = local write "Boolean 45"(TRUE ("Boolean 45")) -> ()
        }
      }
    }
  }
